vi "Write.vi"(8 "error in (no error)":errorcluster, 9 "Value":variant, 10 "Name":string, 11 "TwinCAT ADS in":refnum<class "TwinCAT ADS.lvclass">) -> (0 "error out":errorcluster, 3 "TwinCAT ADS out":refnum<class "TwinCAT ADS.lvclass">)   [LabVIEW 2018, in "TwinCAT ADS.lvclass"]
uses:
  TwinCAT ADS.lvclass
  TwinCAT.Ads
  TwinCAT ADS.lvclass/TwinCAT ADS.ctl
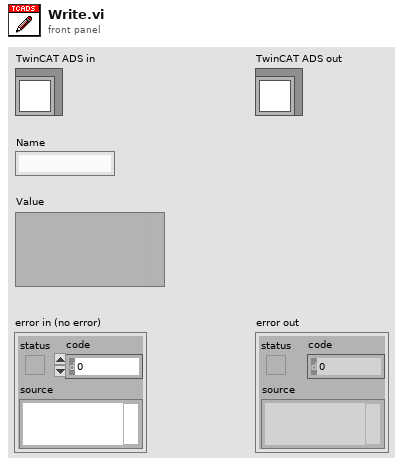
[diagram p1: front panel]
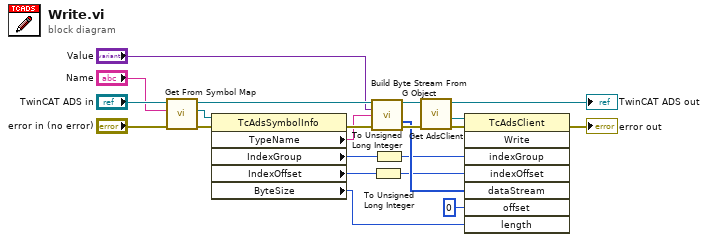
[diagram p0: block diagram]
diagram:
  n1 = call "Get From Symbol Map.vi"("error in (no error)"="error in (no error)", "Symbol Name"="Name", "TwinCAT ADS in"="TwinCAT ADS in") -> ("error out"=w21:errorcluster, ".NET Symbol Information"=w22:refnum<k24>, "TwinCAT ADS out"=w7:refnum<class "TwinCAT ADS.lvclass">)  [unwired: 6 in]
  n2 = property class="TcAdsSymbolInfo"(reference=w22, error in=w21) -> (error out=w9:errorcluster, "TypeName"=w6:string, "IndexGroup"=w14:i64, "IndexOffset"=w15:i64, "ByteSize"=w4:i32)  [unwired: 1 out]
  n3 = call "Build Byte Stream From G Object.vi"("TwinCAT ADS in"=w7, "Value"="Value", "Type Name"=w6, "error in (no error)"=w9) -> ("TwinCAT ADS out"=w10:refnum<class "TwinCAT ADS.lvclass">, "Byte Stream out"=w8:u8[], "error out"=w11:errorcluster)  [unwired: 9 in]
  n4 = To Unsigned Long Integer(number=w15) -> (unsigned 32bit integer=w1:u32)
  n5 = To Unsigned Long Integer(number=w14) -> (unsigned 32bit integer=w2:u32)
  n6 = call "Get AdsClient.vi"("error in (no error)"=w11, "TwinCAT ADS in"=w10) -> ("error out"=w17:errorcluster, ".NET TcAdsClient refnum"=w16:refnum<k24>, "TwinCAT ADS out"=→"TwinCAT ADS out":refnum<class "TwinCAT ADS.lvclass">)  [unwired: 7 in]
  n7 = invoke class="TcAdsClient" method="Write"(reference=w16, error in=w17, "indexGroup"=w2, "indexOffset"=w1, "dataStream"=w8, "offset"=0, "length"=w4) -> (error out=→"error out":errorcluster)  [unwired: 1 in, 7 out]
